vi "GetIntegrationProperties.vi"(8 "error in (no error)":errorcluster, 9 "Channels":T1[](array[typedef]), 10 "Channel Properties":T2[](array[typedef]), 11 "ChannelType":string) -> (0 "error out":errorcluster, 2 "Parent Channel Name":string, 3 "Integration Properties":T4={"Conversion Op"=enum."singleInt", "Unit"="", "Parent Unit"="", "Single Integration Cutoff"=0.0, "Double Integration Cutoff"=0.0, "Lowpass Filter State"={"designed"=FALSE, "integration filter coefficients"={"beta"=0.0, "gamma"=0.0, "alpha"=0.0}, "state"={"x(n-1) state"=0.0, "y(n-1) state"=0.0, "x(n-2) state"=0.0, "y(n-2) state"=0.0}}, "Highpass Filter State"={"designed"=FALSE, "IIR Filter Cluster"={"filter structure"=enum."IIR 2nd Order", "Reverse Coefficients"=[], "Forward Coefficients"=[]}, "Filter State"=[]}, "Wfm Scale"=0.0} {"Highpass Filter State"."Filter State" format="%.2f"; "Highpass Filter State"."IIR Filter Cluster"."Forward Coefficients" format="%.2f"; "Highpass Filter State"."IIR Filter Cluster"."Reverse Coefficients" format="%.2f"; "Lowpass Filter State"."state"."y(n-2) state" format="%.2f"; "Lowpass Filter State"."state"."x(n-2) state" format="%.2f"; "Lowpass Filter State"."state"."y(n-1) state" format="%.2f"; "Lowpass Filter State"."state"."x(n-1) state" format="%.2f"})   [LabVIEW 2017, in "CmsVirtualChannel.lvlib"]
uses:
  <vilib>/addons/InsightCM/Devices/Shared/Cms/CmsVirtualChannel/CmsVirtualChannel.lvlib
  <vilib>/addons/InsightCM/MessageBus/Base/controls/KeyValuePair.ctl
  <vilib>/addons/InsightCM/Devices/Shared/Cms/CmsVirtualChannel/controls/Integration.ctl
  <vilib>/addons/InsightCM/Utilities/Analysis/Shared/controls/ConversionOp.ctl
  <vilib>/addons/InsightCM/Utilities/Analysis/Vibration/controls/LowPassFilterState.ctl
  <vilib>/addons/InsightCM/Utilities/Analysis/Vibration/controls/HighPassFilterState.ctl
  <vilib>/addons/InsightCM/MessageBus/Base/controls/R2_Channel.ctl
  <vilib>/addons/InsightCM/MessageBus/Base/controls/Metric.ctl
  <vilib>/addons/InsightCM/Utilities/PropertyHelpers/PropertyHelpers.lvlib
  <vilib>/addons/InsightCM/Utilities/DeviceModelHelpers/DeviceModelHelpers.lvlib
  <vilib>/addons/InsightCM/Utilities/Analysis/Shared/AnalysisHelper.lvlib
  <vilib>/addons/InsightCM/Utilities/Analysis/Vibration/VibrationAnalysisFunctions.lvlib
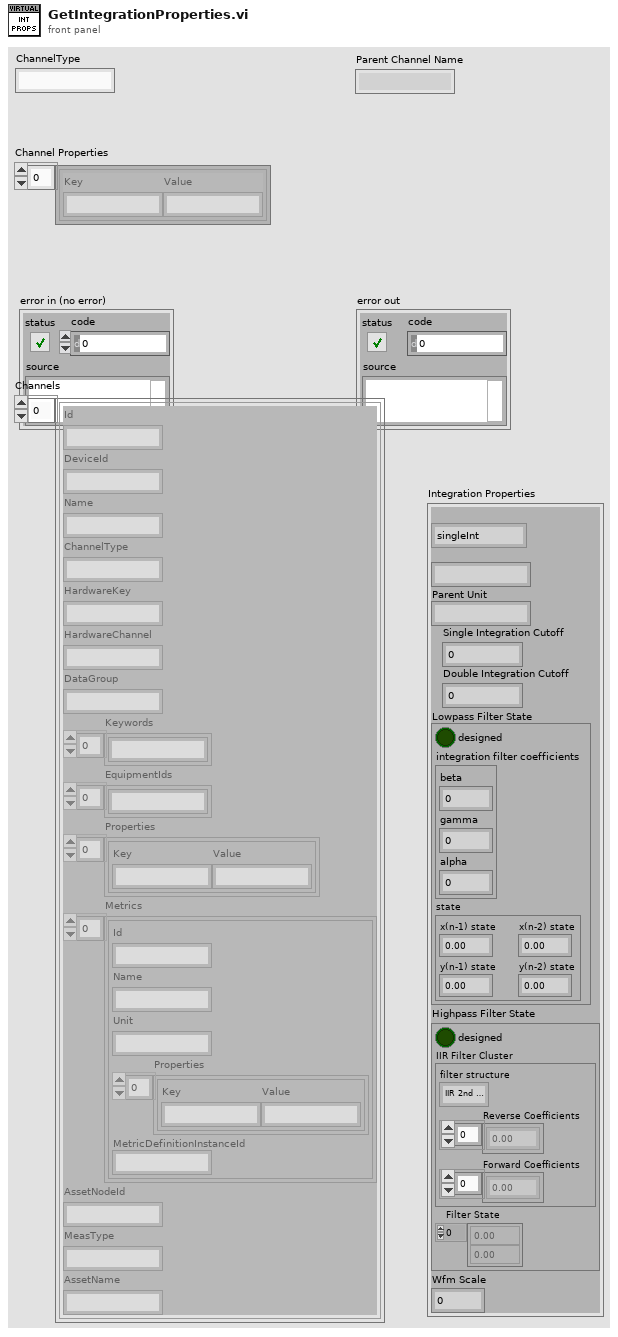
[diagram p1: front panel]
types:
  T1 = typedef "R2_Channel.ctl" = cluster{"Id":string, "DeviceId":string, "Name":string, "ChannelType":string, "HardwareKey":string, "HardwareChannel":string, "DataGroup":string, "Keywords":string[], "EquipmentIds":string[], "Properties":T2[], "Metrics":T3[], "AssetNodeId":string, "MeasType":string, "AssetName":string}
  T2 = typedef "KeyValuePair.ctl" = cluster{"Key":string, "Value":string}
  T3 = typedef "Metric.ctl" = cluster{"Id":string, "Name":string, "Unit":string, "Properties":T2[], "MetricDefinitionInstanceId":string}
  T4 = typedef "CmsVirtualChannel.lvlib/Integration.ctl" = cluster{"Conversion Op":T5, "Unit":string, "Parent Unit":string, "Single Integration Cutoff":dbl, "Double Integration Cutoff":dbl, "Lowpass Filter State":T6, "Highpass Filter State":T7, "Wfm Scale":sgl}
  T5 = typedef "AnalysisHelper.lvlib/ConversionOp.ctl" = enum16{"none", "singleInt", "doubleInt", "singleDiff", "doubleDiff"}
  T6 = typedef "VibrationAnalysisFunctions.lvlib/LowPassFilterState.ctl" = cluster{"designed":bool, "integration filter coefficients":cluster{"beta":dbl, "gamma":dbl, "alpha":dbl}, "state":cluster{"x(n-1) state":dbl, "y(n-1) state":dbl, "x(n-2) state":dbl, "y(n-2) state":dbl}}
  T7 = typedef "VibrationAnalysisFunctions.lvlib/HighPassFilterState.ctl" = cluster{"designed":bool, "IIR Filter Cluster":cluster{"filter structure":enum32{"IIR 2nd Order", "IIR 4th Order"}, "Reverse Coefficients":dbl[], "Forward Coefficients":dbl[]}, "Filter State":dbl[]}
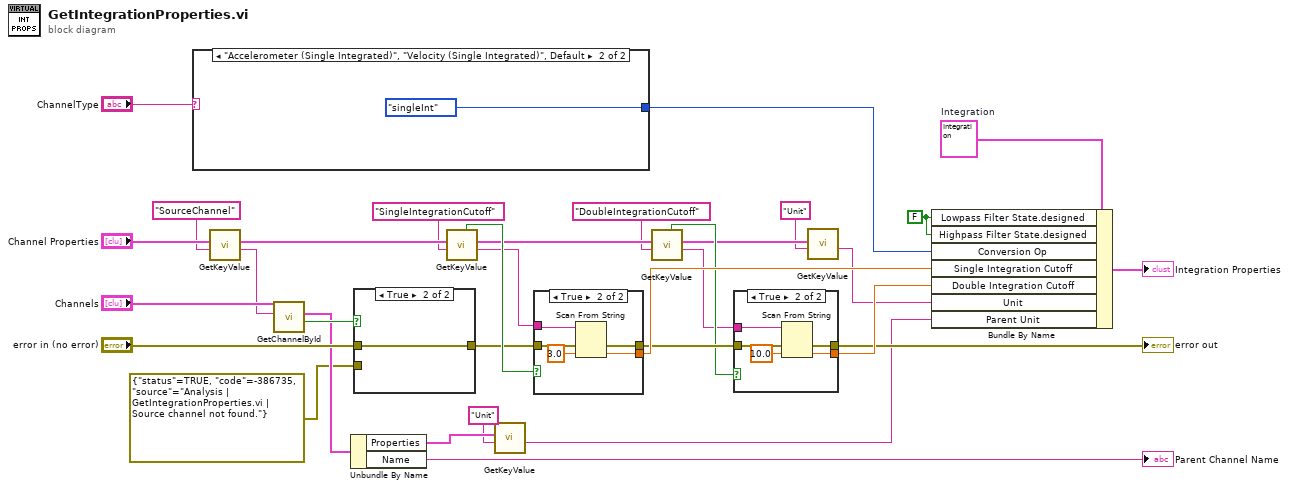
[diagram p0: block diagram]
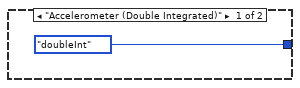
[diagram p2: hidden frame]
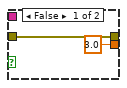
[diagram p4: hidden frame]
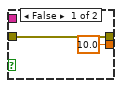
[diagram p5: hidden frame]
diagram:
  w1 = FALSE ("Lowpass Filter State.designed")
  w27 = T4 {"Conversion Op"=enum."singleInt", "Unit"="", "Parent Unit"="", "Single Integration Cutoff"=0.0, "Double Integration Cutoff"=0.0, "Lowpass Filter State"={"designed"=FALSE, "integration filter coefficients"={"beta"=0.0, "gamma"=0.0, "alpha"=0.0}, "state"={"x(n-1) state"=0.0, "y(n-1) state"=0.0, "x(n-2) state"=0.0, "y(n-2) state"=0.0}}, "Highpass Filter State"={"designed"=FALSE, "IIR Filter Cluster"={"filter structure"=enum."IIR 2nd Order", "Reverse Coefficients"=[], "Forward Coefficients"=[]}, "Filter State"=[]}, "Wfm Scale"=0.0}  # Integration
  n1 = case shown="\"Accelerometer (Single Integrated)\", \"Velocity (Single Integrated)\", Default" "ChannelType" {
    tunnel: [ConversionOp."doubleInt" ("Conversion Op") ConversionOp."singleInt" ("Conversion Op")] -> w18
    frame "Accelerometer (Double Integrated)" {
    }
    frame "Accelerometer (Single Integrated)", "Velocity (Single Integrated)", Default {
    }
  }
  n2 = call <vilib>:"GetKeyValue.vi"("key"="SourceChannel" ("name"), "key value pairs"="Channel Properties") -> ("value"=w6:string, "key value pairs out"=w13:T2[])  [unwired: 7 in, 1 out]
  n3 = call <vilib>:"GetChannelById.vi"("channel id"=w6, "channels in"="Channels") -> ("found"=w22:bool, "channel"=w21:T1)  [unwired: 7 in, 1 out]
  n4 = Unbundle By Name(w21) -> ("Properties"=w17:T2[], "Name"=→"Parent Channel Name":string)
  n5 = case shown="True" w22 {
    tunnel: [w36 w37] -> w24
    tunnel: "error in (no error)" -> [_ w37]
    tunnel: errorcluster {"status"=TRUE, "code"=-386735, "source"="Analysis | GetIntegrationProperties.vi | Source channel not found."} ("error in (no error)") -> [w36 _]
    frame False {
    }
    frame True {
    }
  }
  n6 = call <vilib>:"GetKeyValue.vi"("key"="SingleIntegrationCutoff" ("name"), "key value pairs"=w13) -> ("value"=w5:string, "key value pairs out"=w12:T2[], "found"=w28:bool)  [unwired: 7 in]
  n7 = call <vilib>:"GetKeyValue.vi"("key"="Unit" ("name"), "key value pairs"=w17) -> ("value"=w15:string)  [unwired: 7 in, 2 out]
  n8 = case shown="True" w28 {
    tunnel: w5 -> [_ w44]
    tunnel: [3.0 w42] -> w33
    tunnel: w24 -> [w39 w41]
    tunnel: [w39 w40] -> w31
    frame False {
    }
    frame True {
      n9 = Scan From String(input string=w44, error in=w41, default 1=3.0) -> (error out=w40:errorcluster, output 1=w42:dbl)  [unwired: 2 in, 2 out]
    }
  }
  n10 = call <vilib>:"GetKeyValue.vi"("key"="DoubleIntegrationCutoff" ("name"), "key value pairs"=w12) -> ("value"=w4:string, "key value pairs out"=w11:T2[], "found"=w29:bool)  [unwired: 7 in]
  n11 = case shown="True" w29 {
    tunnel: w4 -> [_ w50]
    tunnel: [10.0 w49] -> w32
    tunnel: w31 -> [w46 w48]
    tunnel: [w46 w47] -> w30
    frame False {
    }
    frame True {
      n12 = Scan From String(input string=w50, error in=w48, default 1=10.0) -> (error out=w47:errorcluster, output 1=w49:dbl)  [unwired: 2 in, 2 out]
    }
  }
  "error out" <- w30
  n13 = call <vilib>:"GetKeyValue.vi"("key"="Unit" ("name"), "key value pairs"=w11) -> ("value"=w3:string)  [unwired: 7 in, 2 out]
  n14 = Bundle By Name(cluster=w27, "Lowpass Filter State.designed"=w1, "Highpass Filter State.designed"=w1, "Conversion Op"=w18, "Single Integration Cutoff"=w33, "Double Integration Cutoff"=w32, "Unit"=w3, "Parent Unit"=w15) -> (→"Integration Properties":T4)
